vi "Emballage_BDD_enregistrement_valeur.vi"(6 "SN_PRODUIT":string, 7 "NO_CDEVAL":string, 8 "Error in":errorcluster caption="Error in (no error)", 10 "NO_DU_CARTON":i32, 11 "ID_UTILISATEUR_GPAO":string) -> (0 "Error out":errorcluster)   [LabVIEW 2020]
uses:
  Modules/FS/60_FS_Controles/60_FS_SetGet.ctl
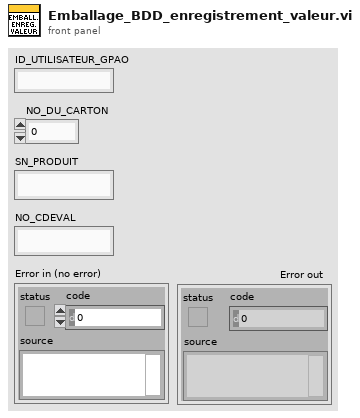
[diagram p1: front panel]
types:
  T1 = typedef "60_FS_SetGet.ctl" = enum16{"set", "get"}
  T2 = typedef "Emballage_BDD_param_Produit.ctl" = cluster{"No_Valve_FAS":string, "suffixe":string, "designation":string, "indice_produit":string, "code_barre_fixe":string, "affiche_code_barre_client":string, "affiche_no_client":string, "Nb_vlve_par_carton":u16, "melange_des_lots_possible":string, "id_article":string, "Indice_Rev":string, "Famille":string, "date":string, "code_barre_fixe_Fin":string, "Longeur_No_Serie":string}
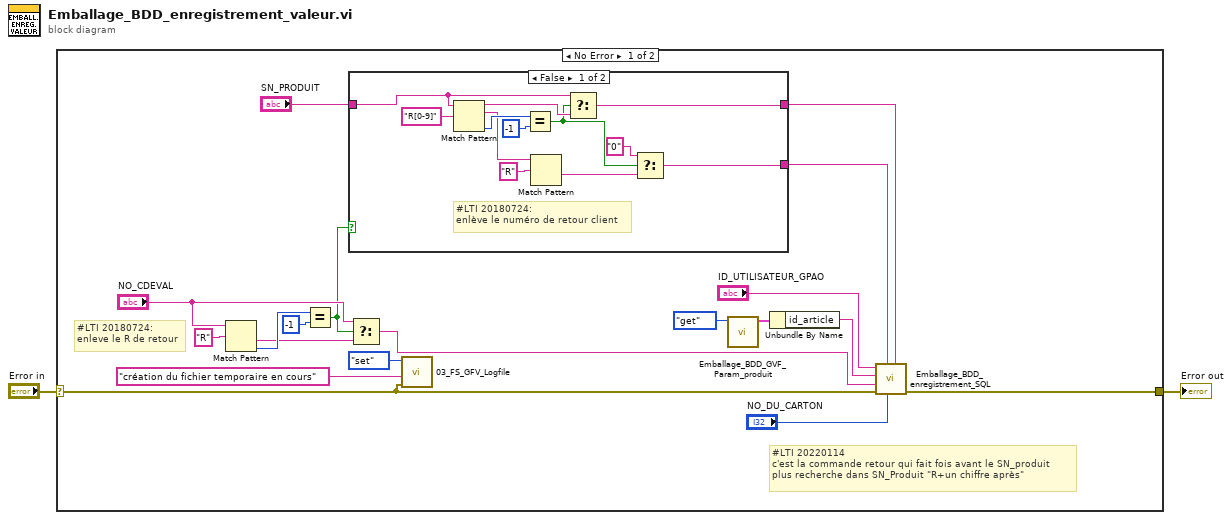
[diagram p0: block diagram]
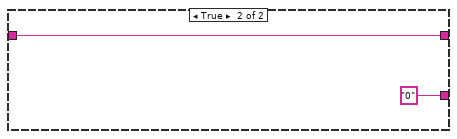
[diagram p2: hidden frame]
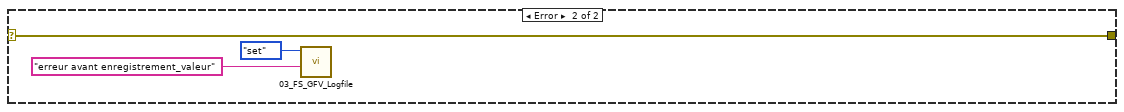
[diagram p3: hidden frame]
diagram:
  n1 = case shown="No Error" "Error in" {
    selector: "Error in" -> [w5 w38]
    tunnel: [w7 w38] -> w1
    frame No Error {
      # "#LTI 20220114\nc'est la commande retour qui fait fois avant le SN_produit\nplus recherche dans SN_Produit \"R+un chiffre après\""
      # "#LTI 20180724:\nenleve le R de retour"
      n2 = Match Pattern(string="NO_CDEVAL", regular expression="R" ("expression régulière")) -> (after substring=w17:string, offset past match=w19:i32)  [unwired: 1 in, 2 out]
      n3 = Equal?(x=w19, y=-1) -> (x = y?=w3:bool)
      n4 = case shown="False" w3 {
        tunnel: "SN_PRODUIT" -> [w28 w35]
        tunnel: [w27 w35] -> w9
        tunnel: [w26 "0" ("SN_PRODUIT")] -> w8
        frame False {
          # "#LTI 20180724:\nenlève le numéro de retour client"
          n5 = Match Pattern(string=w28, regular expression="R[0-9]" ("expression régulière")) -> (before substring=w31:string, match substring=w24:string, offset past match=w32:i32)  [unwired: 1 in, 1 out]
          n6 = Equal?(x=w32, y=-1) -> (x = y?=w25:bool)
          n7 = Match Pattern(string=w24, regular expression="R") -> (after substring=w22:string)  [unwired: 1 in, 3 out]
          n8 = Select(t=w28, s=w25, f=w31) -> (s? t:f=w27:string)
          n9 = Select(t="0" ("expression régulière"), s=w25, f=w22) -> (s? t:f=w26:string)
        }
        frame True {
        }
      }
      n10 = Select(t="NO_CDEVAL", s=w3, f=w17) -> (s? t:f=w16:string)
      n11 = call "03_FS_GFV_Logfile.vi"("error in"=w5, "Chaîne"="création du fichier temporaire en cours", "States"=60_FS_SetGet."set") -> ()  [unwired: 7 in, 2 out]
      n12 = call "Emballage_BDD_GVF_Param_produit.vi"("Énum"=enum16{"set", "get"}."get") -> ("CLS_param_produit"=w14:T2)  [unwired: 7 in, 3 out]
      n13 = Unbundle By Name(w14) -> ("id_article"=w13:string)
      n14 = call "Emballage_BDD_enregistrement_SQL.vi"("SN_PRODUIT"=w9, "NO_DU_CARTON"="NO_DU_CARTON", "NO_RETOUR_CLIENT"=w8, "entrée d'erreur"=w5, "NO_CDEVAL"=w16, "ID_ARTICLE_GPAO"=w13, "ID_UTILISATEUR_GPAO"="ID_UTILISATEUR_GPAO") -> ("sortie d'erreur"=w7:errorcluster)  [unwired: 4 in]
    }
    frame Error {
      n15 = call "03_FS_GFV_Logfile.vi"("Chaîne"="erreur avant enregistrement_valeur", "States"=60_FS_SetGet."set") -> ()  [unwired: 8 in, 2 out]
    }
  }
  "Error out" <- w1
